vi "Max2.vi"(6 "Refnum in":T2, 7 "Search Lines":T3[](array[typedef]) {"Edge Info"."Distance (Real-World)" format="%.2f"; "Edge Info"."Location (Real-World)"."Y" format="%.2g"; "Edge Info"."Location (Real-World)"."X" format="%.2f"; "Edge Info"."Noise" format="%.2f"; "Edge Info"."Location (Pixel)"."Y" format="%.2g"; "Edge Info"."Location (Pixel)"."X" format="%.2f"; "Edge Info"."Strength" format="%.2f"; "Edge Info"."Distance (Pixel)" format="%.2f"}, 9 "Last Edges":T1[](array[typedef]) {"Distance (Real-World)" format="%.2f"; "Location (Real-World)"."Y" format="%.2g"; "Location (Real-World)"."X" format="%.2f"; "Noise" format="%.2f"; "Location (Pixel)"."Y" format="%.2g"; "Location (Pixel)"."X" format="%.2f"; "Strength" format="%.2f"; "Distance (Pixel)" format="%.2f"}, 10 "First Edges":T1[](array[typedef]) {"Distance (Real-World)" format="%.2f"; "Location (Real-World)"."Y" format="%.2g"; "Location (Real-World)"."X" format="%.2f"; "Noise" format="%.2f"; "Location (Pixel)"."Y" format="%.2g"; "Location (Pixel)"."X" format="%.2f"; "Strength" format="%.2f"; "Distance (Pixel)" format="%.2f"}, 11 "Refnum in":T2) -> (2 "Distance":dbl, 3 "Array":cluster{"X":sgl, "Y":sgl}[](array[cluster]))   [LabVIEW 2019, in "Algorithm.lvclass"]
uses:
  FrameworkOverrides/Algorithm.lvclass
  <vilib>/vision/NI_Vision_Development_Module.lvlib
  <vilib>/vision/Measure.llb/Edge Polarity.ctl
  <vilib>/vision/Measure.llb/Edge Options.ctl
  <vilib>/vision/Measure.llb/Straight Edge Process.ctl
  <vilib>/vision/Measure.llb/Straight Edge Options.ctl
  <vilib>/vision/Measure.llb/Edge New.ctl
  <vilib>/vision/Measure.llb/Search Line.ctl
  <vilib>/vision/Image Controls.llb/IMAQ Image.ctl
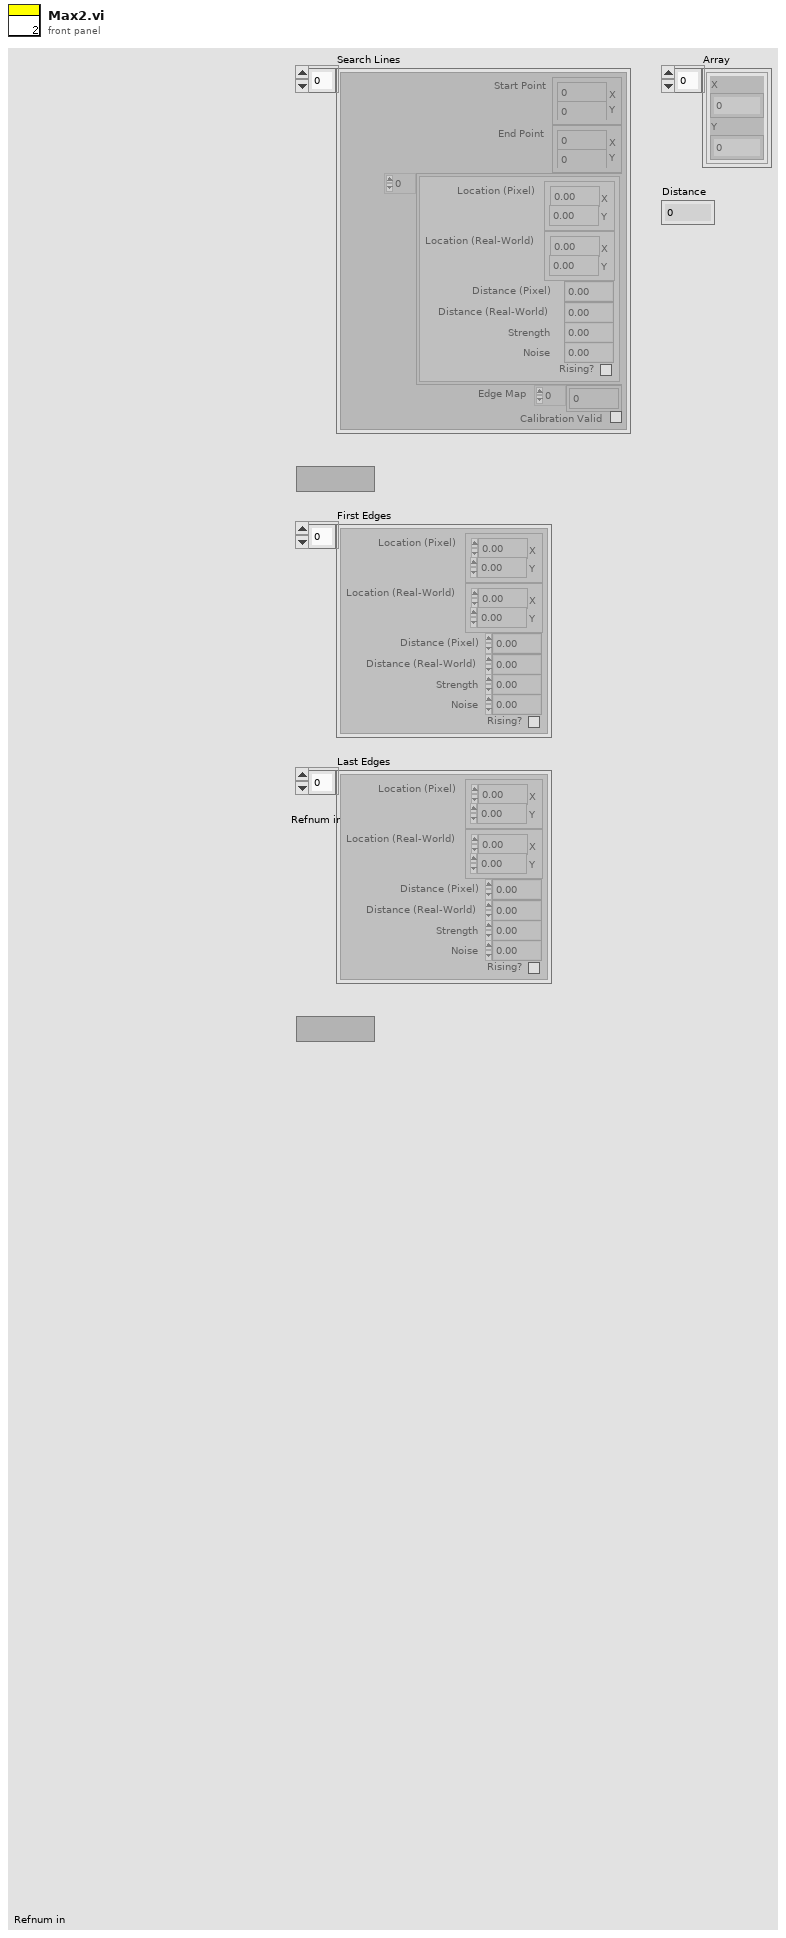
[diagram p1: front panel]
types:
  T1 = typedef "Edge New.ctl" = cluster{"Location (Pixel)":cluster{"X":sgl, "Y":sgl}, "Location (Real-World)":cluster{"X":sgl, "Y":sgl}, "Distance (Pixel)":dbl, "Distance (Real-World)":dbl, "Strength":dbl, "Noise":dbl, "Rising?":bool}
  T2 = typedef "IMAQ Image.ctl" = refnum<image>
  T3 = typedef "Search Line.ctl" = cluster{"Start Point":cluster{"X":sgl, "Y":sgl}, "End Point":cluster{"X":sgl, "Y":sgl}, "Edge Info":T1[], "Edge Map":dbl[], "Calibration Valid":bool}
  T4 = typedef "Straight Edge Options.ctl" = cluster{"Number of Lines":i32, "Type":T5, "Min. Score":dbl, "Max. Score":dbl, "Orientation":dbl, "Angle Range":dbl, "Angle Tolerance":dbl, "Step Size":u32, "Min. SNR (db)":dbl, "Min. Points (%)":dbl, "Hough Iterations":i32}
  T5 = typedef "Straight Edge Process.ctl" = enum32{"First Edge Rake", "Best Edge Rake", "Hough Edge Rake", "First Edge Projection", "Best Edge Projection"}
  T6 = typedef "Edge Options.ctl" = cluster{"Edge Polarity":T7, "Kernel Size":u32, "Width":u32, "Minimum Edge Strength":sgl, "Interpolation Type":enum32{"Zero Order", "Bilinear", "Quadratic", "Cubic", "Bilinear Fixed"}, "Data Processing Method":enum32{"Average", "Median"}}
  T7 = typedef "Edge Polarity.ctl" = u32
  T8 = typedef "IMAQ Rectangle" = cluster{"Left":i32, "Top":i32, "Right":i32, "Bottom":i32, "Rotation":dbl}
  T9 = cluster{"Point 1":cluster{"X":sgl, "Y":sgl}, "Point 2":cluster{"X":sgl, "Y":sgl}}
  T10 = typedef "ROI Descriptor" = cluster{"Global Rectangle":i32[], "Contours":cluster{"ID":enum32{"External", "Internal"}, "Type":u32, "Coordinates":i32[]}[]}
  T11 = cluster{"Point1 (Pixels)":cluster{"X":sgl, "Y":sgl}, "Point2 (Pixels)":cluster{"X":sgl, "Y":sgl}, "Point1 (Real-World)":cluster{"X":sgl, "Y":sgl}, "Point2 (Real-World)":cluster{"X":sgl, "Y":sgl}, "Angle (Pixel)":dbl, "Angle (Real-World)":dbl, "Score":dbl, "Straightness":dbl, "Average SNR (db)":dbl, "Calibration Valid":bool}[]
  T12 = cluster{"Point1 (Pixels)":cluster{"X":sgl, "Y":sgl}, "Point2 (Pixels)":cluster{"X":sgl, "Y":sgl}, "Point1 (Real-World)":cluster{"X":sgl, "Y":sgl}, "Point2 (Real-World)":cluster{"X":sgl, "Y":sgl}, "Angle (Pixel)":dbl, "Angle (Real-World)":dbl, "Score":dbl, "Straightness":dbl, "Average SNR (db)":dbl, "Calibration Valid":bool}
  T13 = cluster{"Start Point":cluster{"X":sgl, "Y":sgl}, "Location (Pixel)":cluster{"X":sgl, "Y":sgl}, "Point 2":cluster{"X":sgl, "Y":sgl}, "Point 2":cluster{"X":sgl, "Y":sgl}}
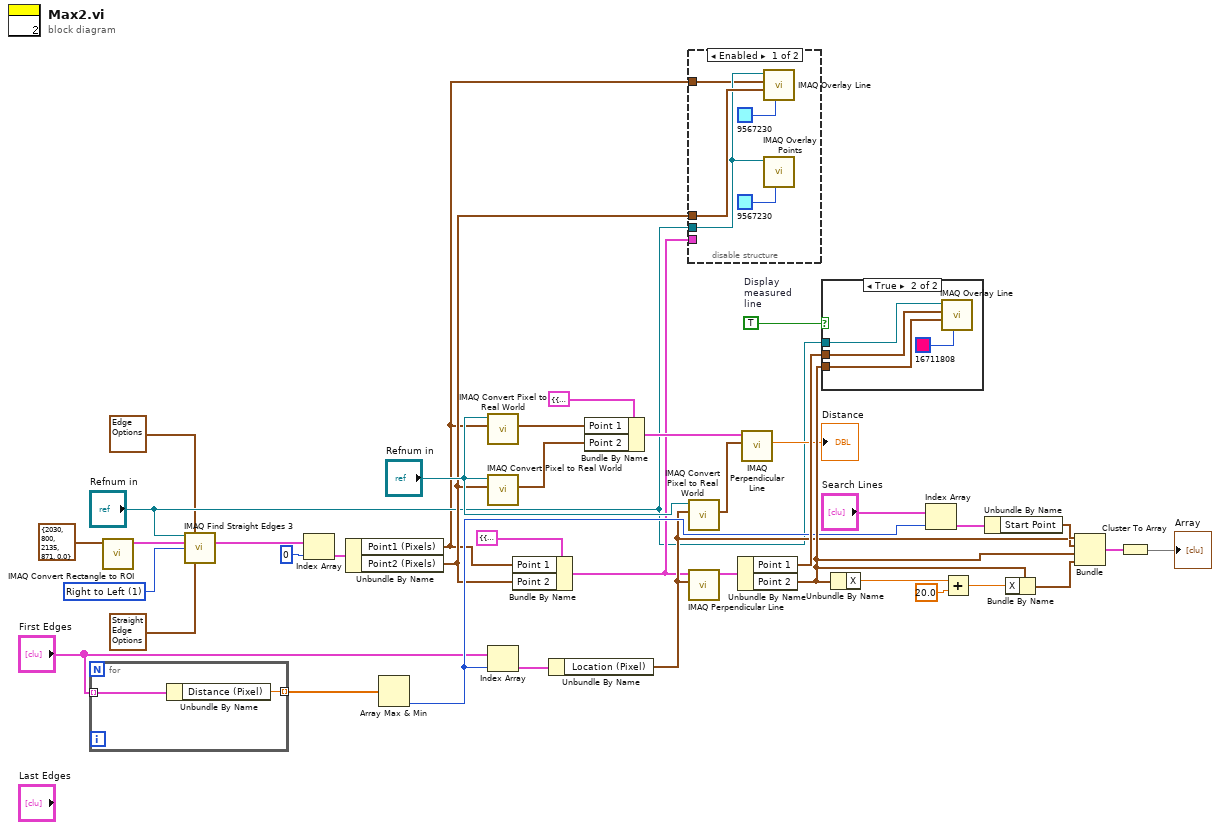
[diagram p0: block diagram]
diagram:
  w5 = u32 1 items=["Left to Right", "Right to Left", "Top to Bottom", "Bottom to Top"] ("Search Direction")
  w38 = TRUE  # Display  measured line
  n1 = for {
    tunnel: "First Edges" -> [w40] mode=indexing
    tunnel: [w39] -> w16 mode=indexing
    n2 = Unbundle By Name(w40) -> ("Distance (Pixel)"=w39:dbl)
  }
  n3 = call "IMAQ Convert Rectangle to ROI"("Rectangle"=T8 {"Left"=2030, "Top"=800, "Right"=2135, "Bottom"=871, "Rotation"=0.0}) -> ("ROI Descriptor"=w7:T10)  [unwired: 8 in, 1 out]
  n4 = call "IMAQ Find Straight Edges 3"("Image"="Refnum in", "Edge Options"=T6 {"Edge Polarity"=2, "Kernel Size"=3, "Width"=3, "Minimum Edge Strength"=50.0, "Interpolation Type"=enum."Zero Order", "Data Processing Method"=enum."Average"}, "ROI Descriptor"=w7, "Search Direction"=w5, "Line Options"=T4 {"Number of Lines"=1, "Type"=enum."First Edge Rake", "Min. Score"=500.0, "Max. Score"=1000.0, "Orientation"=0.0, "Angle Range"=1.0, "Angle Tolerance"=1.0, "Step Size"=5, "Min. SNR (db)"=0.0, "Min. Points (%)"=25.0, "Hough Iterations"=5}) -> ("Straight Edges"=w14:T11)  [unwired: 6 in, 4 out]
  n5 = Index Array(array=w14, index=0) -> (element=w13:T12)
  n6 = Unbundle By Name(w13) -> ("Point1 (Pixels)"=w3:cluster{"X":sgl, "Y":sgl}, "Point2 (Pixels)"=w10:cluster{"X":sgl, "Y":sgl})
  n7 = Array Max & Min(array=w16) -> (min index (indices)=w28:i32)  [unwired: 3 out]
  n8 = call "IMAQ Convert Pixel to Real World"("Pixel Coordinates"=w3, "Calibrated Image"="Refnum in") -> ("Real World Coordinates"=w22:cluster{"X":sgl, "Y":sgl})  [unwired: 4 in, 5 out]
  n9 = call "IMAQ Convert Pixel to Real World"("Pixel Coordinates"=w10, "Calibrated Image"="Refnum in") -> ("Real World Coordinates"=w24:cluster{"X":sgl, "Y":sgl})  [unwired: 4 in, 5 out]
  n10 = Index Array(array="First Edges", index=w28) -> (element=w18:T1)
  n11 = Bundle By Name(cluster=T9 {"Point 1"={"X"=0.0, "Y"=0.0}, "Point 2"={"X"=0.0, "Y"=0.0}} ("Line Segment"), "Point 1"=w3, "Point 2"=w10) -> (w9:T9)
  n12 = Unbundle By Name(w18) -> ("Location (Pixel)"=w15:cluster{"X":sgl, "Y":sgl})
  n13 = Bundle By Name(cluster=T9 {"Point 1"={"X"=0.0, "Y"=0.0}, "Point 2"={"X"=0.0, "Y"=0.0}} ("Line"), "Point 1"=w22, "Point 2"=w24) -> (w25:T9)
  n14 = disable-structure shown="Enabled" {
    disable-tunnel: w9 -> [_ _]
    disable-tunnel: w10 -> [w45 _]
    disable-tunnel: "Refnum in" -> [w44 _]
    disable-tunnel: w3 -> [w41 _]
    frame Enabled {
      n15 = call "IMAQ Overlay Line"("Color"=u32 9567230, "End Point"=w45, "Start Point"=w41, "Image"=w44) -> ()  [unwired: 6 in, 2 out]
      n16 = call "IMAQ Overlay Points"("Color"=u32 9567230, "Image"=w44) -> ()  [unwired: 8 in, 2 out]
    }
    frame Disabled {
    }
  }
  n17 = call "IMAQ Convert Pixel to Real World"("Pixel Coordinates"=w15, "Calibrated Image"="Refnum in") -> ("Real World Coordinates"=w19:cluster{"X":sgl, "Y":sgl})  [unwired: 4 in, 5 out]
  n18 = call "IMAQ Perpendicular Line"("Point"=w15, "Line"=w9) -> ("Perpendicular Line"=w26:T9)  [unwired: 7 in, 2 out]
  n19 = Unbundle By Name(w26) -> ("Point 1"=w31:cluster{"X":sgl, "Y":sgl}, "Point 2"=w33:cluster{"X":sgl, "Y":sgl})
  n20 = call "IMAQ Perpendicular Line"("Point"=w19, "Line"=w25) -> ("Distance"=→"Distance":dbl)  [unwired: 7 in, 2 out]
  n21 = case shown="True" w38 {
    tunnel: "Refnum in" -> [_ w49]
    tunnel: w31 -> [_ w47]
    tunnel: w33 -> [_ w46]
    frame False {
    }
    frame True {
      n22 = call "IMAQ Overlay Line"("Color"=u32 16711808, "End Point"=w46, "Start Point"=w47, "Image"=w49) -> ()  [unwired: 6 in, 2 out]
    }
  }
  n23 = Unbundle By Name(w33) -> ("X"=w34:sgl)
  n24 = Index Array(array="Search Lines", index=w28) -> (element=w29:T3)
  n25 = Add(x=w34, y=sgl 20.0) -> (x+y=w36:sgl)
  n26 = Unbundle By Name(w29) -> ("Start Point"=w30:cluster{"X":sgl, "Y":sgl})
  n27 = Bundle By Name(cluster=w33, "X"=w36) -> (w37:cluster{"X":sgl, "Y":sgl})
  n28 = Bundle("Start Point"=w30, "Location (Pixel)"=w15, "Point 2"=w33, "Point 2"=w37) -> (w32:T13)  [unwired: 1 in]
  n29 = Cluster To Array(cluster=w32) -> (array=→"Array":cluster{"X":sgl, "Y":sgl}[])
